vi "svm_get_libsvm_version.vi"(8 "error in (no error)":errorcluster) -> (0 "error out":errorcluster, 3 "version":i32)   [LabVIEW 2015]
uses:
  bin/LabVIEW-libsvm.so
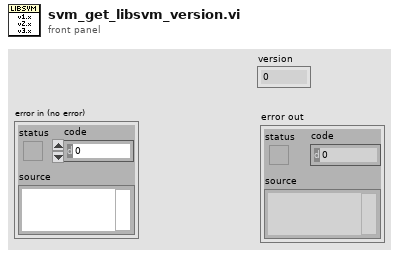
[diagram p1: front panel]
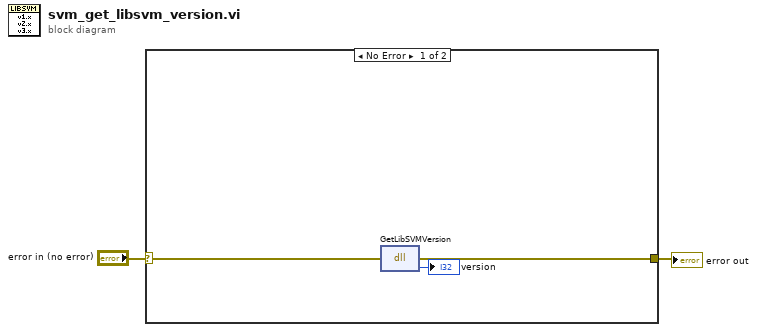
[diagram p0: block diagram]
diagram:
  n1 = case shown="No Error" "error in (no error)" {
    selector: "error in (no error)" -> [w5 w6]
    tunnel: [w3 w6] -> w2
    frame No Error {
      n2 = dll-call lib="home/os/dev/LabVIEW-libsvm/LabVIEW/bin/LabVIEW-libsvm.so" fn="GetLibSVMVersion"(error in=w5) -> (error out=w3:errorcluster, "return type"=→"version":i32)  [unwired: 2 in, 1 out]
    }
    frame Error {
    }
  }
  "error out" <- w2
